vi "Array to CatStr.vi"   [LabVIEW 2019]
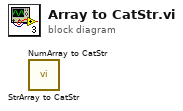
[diagram p0: block diagram]
diagram:
  n1 = call "StrArray to CatStr.vi"() -> ()  [unwired: 1 in, 1 out]
  n2 = call "NumArray to CatStr.vi"() -> ()  [unwired: 1 in, 1 out]
